vi "xiCam - Get1DImageData.vi"(7 "timeout":i32, 8 "error in (no error)":errorcluster, 9 "1DImageData In":u8[](array[numeric]), 10 "input cluster":T1={"WIDTH"=4704, "HEIGHT"=3424, "IMG_FORMAT"=enum."MONO8"}, 11 "xiCam In":refnum<k24>) -> (0 "error out":errorcluster, 1 "1DImageData Out":u8[](array[numeric]), 3 "xiCam Out":refnum<k24>, 4 "Image Properites":T1)   [LabVIEW 2018]
doc: "This function acquires image and returns a preallocated byte array containing the Image data.\n\n<b>void GetImage(byte* ImageData, int timeout)</b>\nint timeout : Time interval required to wait for the image (in milliseconds)"
uses:
  D:/codes labview/VisionLibrariesXimea/xiLib/xiLIB_64bit/xiLIB/xiCamLib/API/x64/xiApi.NETX64.dll
  API/x64/xiApi.NETX64.dll
  Utils/xiImageManager/xiImageMng - Attributes.ctl
  PRM/IMG_FORMAT/IMG_DATA_FORMAT.ctl
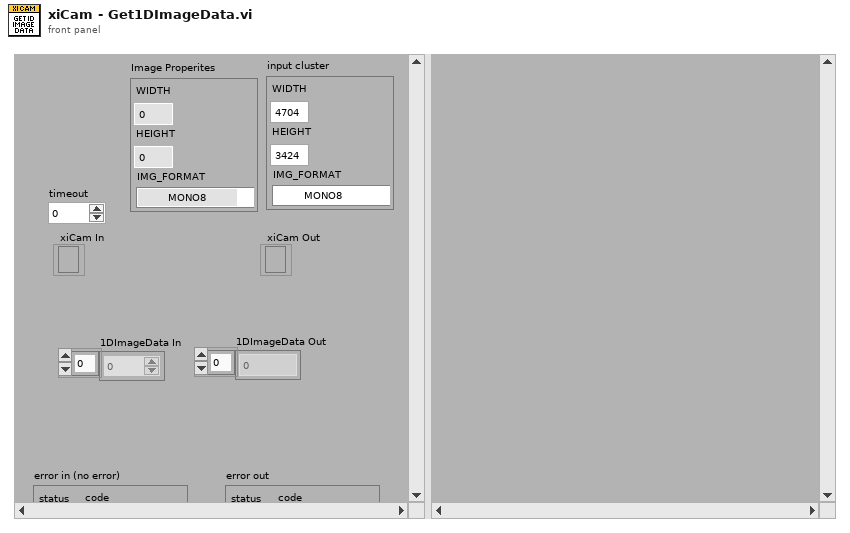
[diagram p1: front panel]
types:
  T1 = typedef "xiImageMng - Attributes.ctl" = cluster{"WIDTH":i32, "HEIGHT":i32, "IMG_FORMAT":T2}
  T2 = typedef "IMG_DATA_FORMAT.ctl" = enum16{"MONO8", "MONO16", "RGB24", "RGB32", "RGBPLANAR", "RAW8", "RAW16"}
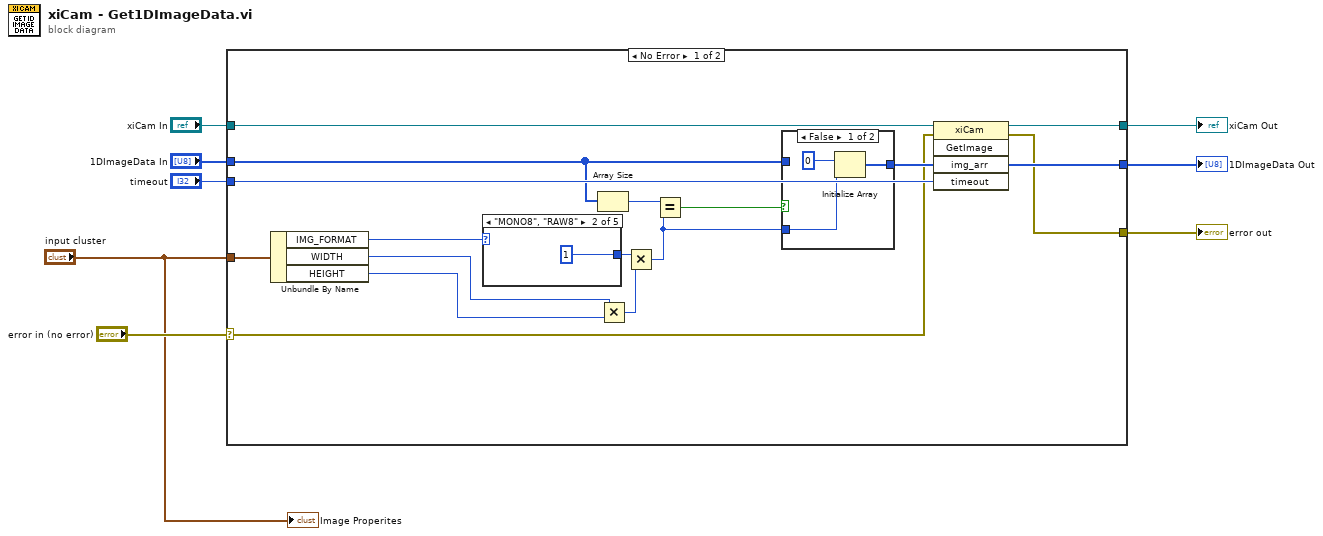
[diagram p0: block diagram]
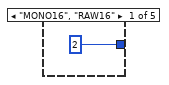
[diagram p2: hidden frame]
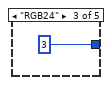
[diagram p3: hidden frame]
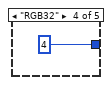
[diagram p4: hidden frame]
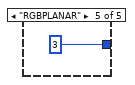
[diagram p5: hidden frame]
diagram:
  n1 = case shown="No Error" "error in (no error)" {
    selector: "error in (no error)" -> [w10 w35]
    tunnel: "xiCam In" -> [w25 w36]
    tunnel: [w24 w36] -> w6
    tunnel: [w21 w35] -> w5
    tunnel: "timeout" -> [w23 _]
    tunnel: [w22 _] -> w3
    tunnel: "1DImageData In" -> [w16 _]
    tunnel: "input cluster" -> [w9 _]
    frame No Error {
      n2 = Unbundle By Name(w9) -> ("IMG_FORMAT"=w12:T2, "WIDTH"=w20:i32, "HEIGHT"=w19:i32)
      n3 = case shown="\"MONO8\", \"RAW8\"" w12 {
        tunnel: [2 ("x*y") 1 ("x*y") 3 ("x*y") 4 ("x*y") 3 ("x*y")] -> w11
        frame "MONO16", "RAW16" {
        }
        frame "MONO8", "RAW8" {
        }
        frame "RGB24" {
        }
        frame "RGB32" {
        }
        frame "RGBPLANAR" {
        }
      }
      n4 = Array Size(array=w16) -> (size(s)=w18:i32)
      n5 = Multiply(x=w20, y=w19) -> (x*y=w14:i32)
      n6 = Multiply(x=w11, y=w14) -> (x*y=w13:i32)
      n7 = Equal?(x=w18, y=w13) -> (x = y?=w17:bool)
      n8 = case shown="False" w17 {
        tunnel: w16 -> [_ w34]
        tunnel: [w31 w34] -> w15
        tunnel: w13 -> [w32 _]
        frame False {
          n9 = Initialize Array(u8 0, w32) -> (w31:u8[])
        }
        frame True {
        }
      }
      n10 = invoke class="xiCam" method="GetImage"(reference=w25, error in=w10, "img_arr"=w15, "timeout"=w23) -> (reference out=w24:refnum<k24>, error out=w21:errorcluster, "img_arr"=w22:u8[])  [unwired: 1 in, 2 out]
    }
    frame Error {
    }
  }
  "error out" <- w5
  "xiCam Out" <- w6
  "1DImageData Out" <- w3
  "Image Properites" <- "input cluster"
